vi "CLSUIP_Get Unwired Terminal of Node.vi"(4 "error in":errorcluster, 7 "NmdBundler Ref":refnum<vi>) -> (0 "error out":errorcluster, 1 "Term Refnum":refnum<vi>, 3 "NmdBundler Ref out":refnum<vi>)   [LabVIEW 2021, in "MemberVICreation.lvlib" / "ElementWrapperRetooler.lvclass"]
uses:
  <resource>/Framework/Providers/LVClassLibrary/NewAccessors/ElementWrapperRetooler/ElementWrapperRetooler.lvclass
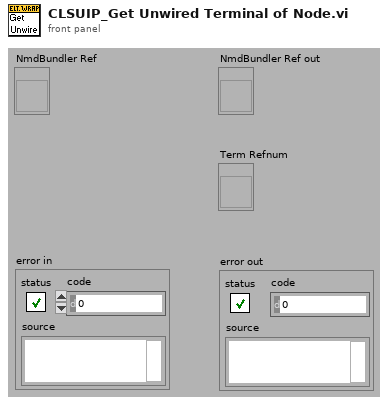
[diagram p1: front panel]
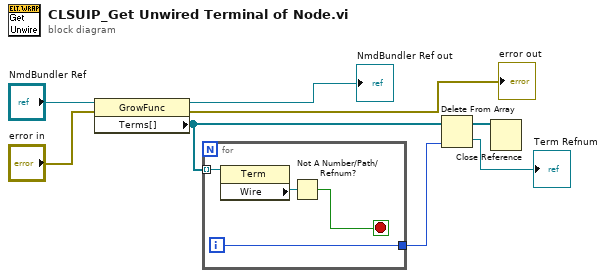
[diagram p0: block diagram]
diagram:
  n1 = property on="Property Node" class="GrowFunc"(reference="NmdBundler Ref", error in="error in") -> (reference out=→"NmdBundler Ref out":refnum<vi>, error out=→"error out":errorcluster, "Terms[]"=w5:refnum<vi>[])
  n2 = for {
    tunnel: w5 -> [w12] mode=indexing
    tunnel: [w9] -> w4
    i -> [w9]
    stop <- w11 stop-if-true
    n3 = property on="Property Node" class="Term"(reference=w12) -> ("Wire"=w10:refnum<vi>)  [unwired: 1 in, 2 out]
    n4 = Not A Number/Path/Refnum?(number/path/refnum=w10) -> (NaN/Path/Refnum?=w11:bool)
  }
  n5 = Delete From Array(array=w5, index=w4) -> (deleted portion=→"Term Refnum":refnum<vi>, array with subset deleted=w3:refnum<vi>[])  [unwired: 1 in]
  n6 = Close Reference(reference=w3) -> ()  [unwired: 1 in, 1 out]
